vi "Setup subWorker - Modbus PLC.vi"(8 "error in":errorcluster, 11 "gui in":refnum<class "gui.lvclass">) -> (0 "error out":errorcluster, 3 "gui out":refnum<class "gui.lvclass">)   [LabVIEW 2023, in "GUI.lvlib" / "gui.lvclass"]
doc: "This VI sets up the framework parameters of a statically-linked subWorker."
uses:
  gui.lvclass
  gui.lvclass/gui.ctl
  Modbus PLC/Modbus PLC/Modbus PLC.lvclass
  J:/Work/Cortech/KTM 1001/Workers Hardware/Workers/Base Classes/Base Hardware/Base Hardware.lvclass
  C:/Program Files/National Instruments/LabVIEW 2023/vi.lib/addons/_Workers/Library/Classes/Worker/Worker.lvclass
  C:/Program Files/National Instruments/LabVIEW 2023/vi.lib/addons/_Workers/Library/Classes/Workers Object/Workers Object.lvclass
  J:/Work/Cortech/KTM 1001/Workers Hardware/Hardware Interface/Hardware Interface.lvclass
  J:/Work/Cortech/KTM 1001/Modbus PLC/Modbus PLC/Modbus PLC.lvclass
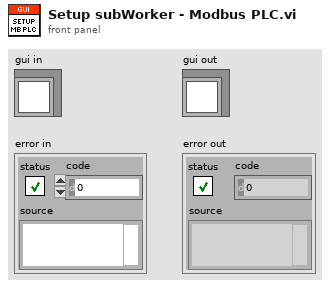
[diagram p1: front panel]
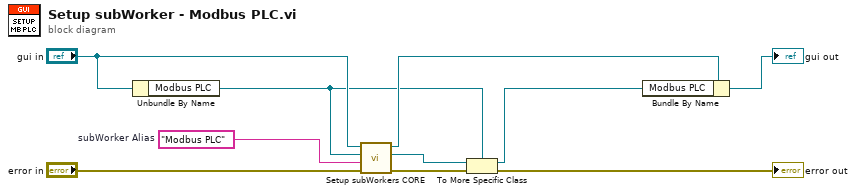
[diagram p0: block diagram]
diagram:
  w6 = "Modbus PLC"  # subWorker Alias
  n1 = Unbundle By Name("gui in") -> ("Modbus PLC"=w3:refnum<class "Modbus PLC.lvclass">)
  n2 = call-dynamic "Setup subWorkers CORE.vi"("error in"="error in", "subWorker Alias"=w6, "subWorker"=w3, "Worker"="gui in") -> ("error out"=w5:errorcluster, "subWorker out"=w1:refnum<class "Worker.lvclass">, "Worker out"=w8:refnum<class "gui.lvclass">)  [unwired: 5 in]
  n3 = To More Specific Class(target class=w3, reference=w1, error in=w5) -> (specific class reference=w2:refnum<class "Modbus PLC.lvclass">, error out=→"error out":errorcluster)
  n4 = Bundle By Name(cluster=w8, "Modbus PLC"=w2) -> (→"gui out":refnum<class "gui.lvclass">)
